vi "Save File.vi"(8 "error in (no error)":errorcluster, 10 "Item Configurations":refnum<class "Item Configuration.lvclass">[](array[class]), 11 "File Path":path) -> (0 "error out":errorcluster)   [LabVIEW 2013, in "File IO.lvlib"]
uses:
  File IO.lvlib
  Item Configuration/Item Configuration/Item Configuration.lvclass
  <vilib>/xml/Load XML File.vi
  <vilib>/xml/Close Reference(Node).vi
  <vilib>/xml/NI_XML.lvlib
  <resource>/objmgr/DOMUserDefRef.rc
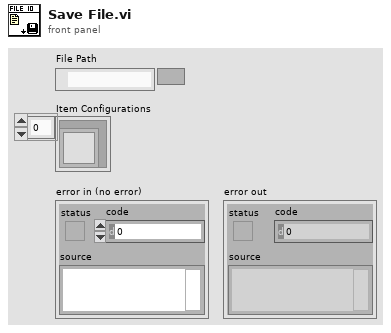
[diagram p1: front panel]
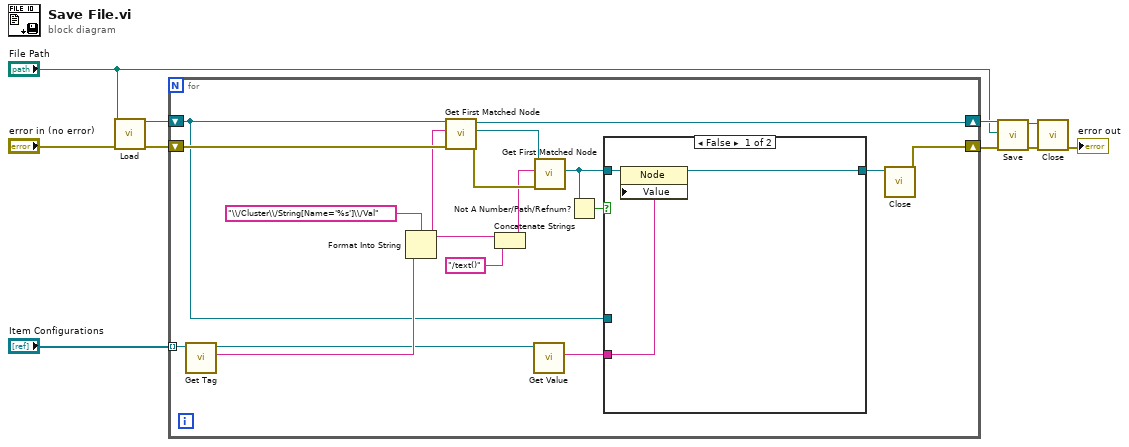
[diagram p0: block diagram]
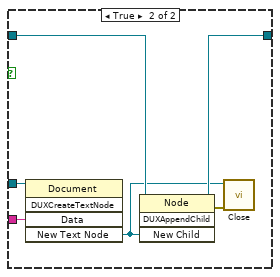
[diagram p2: hidden frame]
diagram:
  n1 = call-poly <vilib>:"Load.vi"("path to XML document"="File Path", "error in (no error)"="error in (no error)") -> ("DOM document out"=w10:refnum<k20>, "error out"=w9:errorcluster)  [unwired: 11 in, 1 out]
  n2 = for {
    shift-right: [w27] -> w5
    shift-left: w10 -> [w12]
    shift-right: [w19] -> w8
    shift-left: w9 -> [w26]
    tunnel: "Item Configurations" -> [w23] mode=indexing
    n3 = call-dynamic "Get Tag.vi"("Item Configuration in"=w23) -> ("Project Info Tag"=w24:string, "Item Configuration out"=w20:refnum<class "Item Configuration.lvclass">)  [unwired: 8 in, 1 out]
    n4 = Format Into String(format string="\\/Cluster\\/String[Name='%s']\\/Val" ("XPath expression"), w24) -> (resulting string=w18:string)  [unwired: 2 in, 1 out]
    n5 = call <vilib>:"Get First Matched Node.vi"("error in (no error)"=w26, "XPath expression"=w18, "node in"=w12) -> ("error out"=w21:errorcluster, "node result"=w22:refnum<k20>, "node out"=w27:refnum<k20>)  [unwired: 6 in]
    n6 = Concatenate Strings(w18, "/text()" ("XPath expression")) -> (w16:string)
    n7 = call-dynamic "Get Value.vi"("Item Configuration in"=w20) -> ("Project Info Value"=w13:string)  [unwired: 8 in, 2 out]
    n8 = call <vilib>:"Get First Matched Node.vi"("error in (no error)"=w21, "XPath expression"=w16, "node in"=w22) -> ("node result"=w14:refnum<k20>)  [unwired: 6 in, 2 out]
    n9 = Not A Number/Path/Refnum?(number/path/refnum=w14) -> (NaN/Path/Refnum?=w15:bool)
    n10 = case shown="False" w15 {
      tunnel: w14 -> [w30 w34]
      tunnel: w13 -> [w28 w36]
      tunnel: w12 -> [_ w35]
      tunnel: [w29 w33] -> w11
      frame False {
        n11 = property class="Node"(reference=w30, "Value"=w28) -> (reference out=w29:refnum<k20>)  [unwired: 1 in, 1 out]
      }
      frame True {
        n12 = invoke class="Document" method="DUXCreateTextNode"(reference=w35, "Data"=w36) -> ("New Text Node"=w31:refnum<k20>)  [unwired: 3 in, 4 out]
        n13 = invoke class="Node" method="DUXAppendChild"(reference=w34, "New Child"=w31) -> (reference out=w33:refnum<k20>, error out=w32:errorcluster)  [unwired: 2 in, 2 out]
        n14 = call-poly <vilib>:"Close.vi"("error in (no error)"=w32, "node"=w31) -> ()  [unwired: 7 in, 1 out]
      }
    }
    n15 = call-poly <vilib>:"Close.vi"("node"=w11) -> ("error out"=w19:errorcluster)  [unwired: 8 in]
  }
  n16 = call <vilib>:"Save.vi"("error in (no error)"=w8, "XML file path"="File Path", "DOM document in"=w5) -> ("error out"=w6:errorcluster, "DOM document out"=w4:refnum<k20>)  [unwired: 6 in, 1 out]
  n17 = call-poly <vilib>:"Close.vi"("error in (no error)"=w6, "node"=w4) -> ("error out"=→"error out":errorcluster)  [unwired: 7 in]
